vi "Functional Global_QRD.vi"(7 "QRD":T1, 8 "error in":errorcluster, 11 "Function":enum16{"Set", "Get"}(ring)=enum."Get") -> (0 "error out":errorcluster, 5 "QRD Out":T1)   [LabVIEW 2025]
uses:
  Controls/Queues-Refs-Data.ctl
  Builds/Queue Wrappers.lvlibp/Q Packet.ctl
  Builds/Queue Wrappers.lvlibp
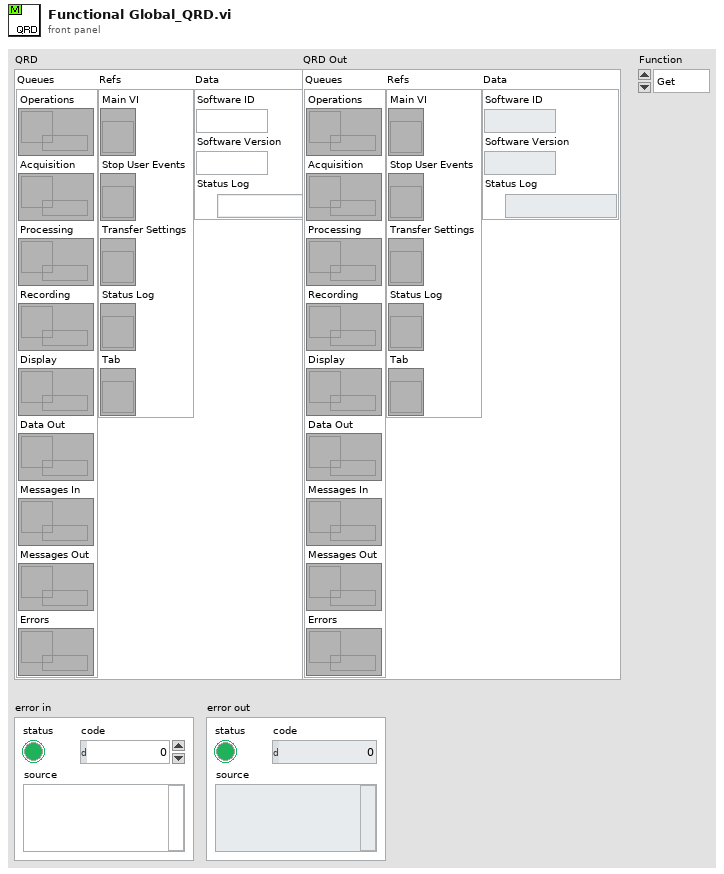
[diagram p1: front panel]
types:
  T1 = typedef "Queues-Refs-Data.ctl" = cluster{"Queues":cluster{"Operations":refnum<queue>, "Acquisition":refnum<queue>, "Processing":refnum<queue>, "Recording":refnum<queue>, "Display":refnum<queue>, "Data Out":refnum<queue>, "Messages In":refnum<queue>, "Messages Out":refnum<queue>, "Errors":refnum<queue>}, "Refs":cluster{"Main VI":refnum<vi>, "Stop User Events":refnum<vi>, "Transfer Settings":refnum<vi>, "Status Log":refnum<vi>, "Tab":refnum<vi>}, "Data":cluster{"Software ID":string, "Software Version":string, "Status Log":path}}
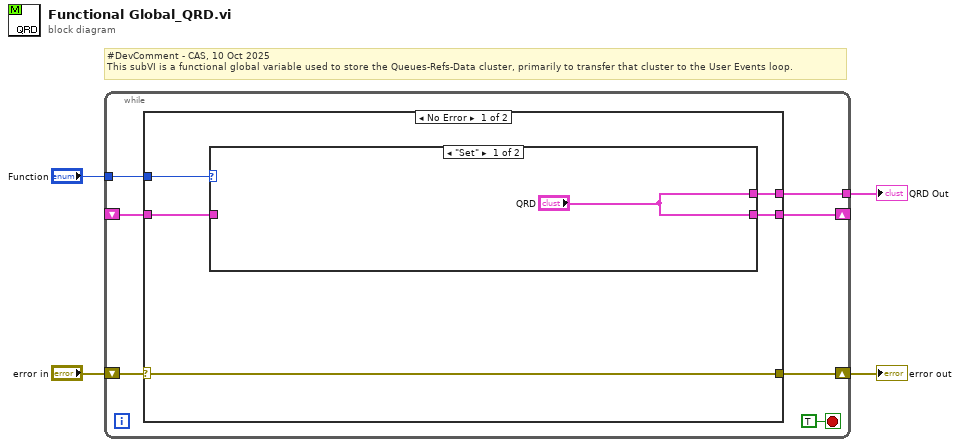
[diagram p0: block diagram]
diagram:
  # "#DevComment - CAS, 10 Oct 2025\nThis subVI is a functional global variable used to store the Queues-Refs-Data cluster, primarily to transfer that cluster to the User Events loop."
  n1 = while {
    shift-right: [w9] -> w1
    shift-left: "error in" -> [w10]
    tunnel: "Function" -> [w8]
    shift-right: [w5] -> _
    shift-left: _ -> [w7]
    tunnel: [w6] -> w2
    stop <- TRUE stop-if-true
    n2 = case shown="No Error" w10 {
      selector: w10 -> [w12 w19]
      tunnel: [w12 w19] -> w9
      tunnel: w8 -> [w16 _]
      tunnel: w7 -> [w15 w20]
      tunnel: [w14 w20] -> w6
      tunnel: [w13 w20] -> w5
      frame No Error {
        n3 = case shown="\"Set\"" w16 {
          tunnel: w15 -> [_ w18]
          tunnel: ["QRD" w18] -> w14
          tunnel: ["QRD" w18] -> w13
          frame "Set" {
          }
          frame "Get", Default {
          }
        }
      }
      frame Error {
      }
    }
  }
  "QRD Out" <- w2
  "error out" <- w1
